vi "tm_setmultiregion_40.vi"(8 "error in (no error)":errorcluster, 10 "Sub Regions":T1(array[cluster]), 11 "Handle in":u32) -> (0 "error out":errorcluster, 3 "Handle out":u32)   [LabVIEW 2023]
uses:
  tmcamcon.dll
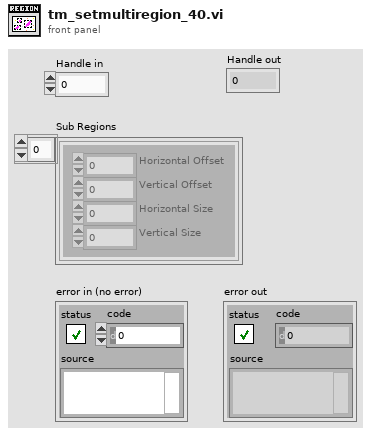
[diagram p1: front panel]
types:
  T1 = cluster{"Horizontal Offset":i32, "Vertical Offset":i32, "Horizontal Size":i32, "Vertical Size":i32}[]
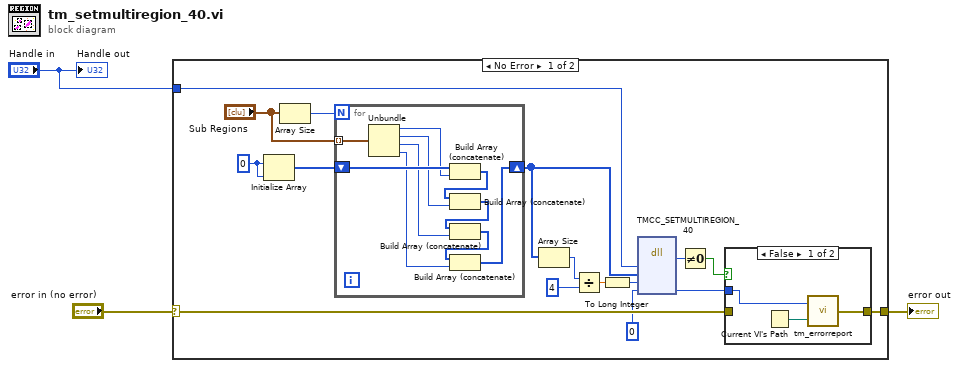
[diagram p0: block diagram]
diagram:
  n1 = case shown="No Error" "error in (no error)" {
    selector: "error in (no error)" -> [w17 w34]
    tunnel: [w14 w34] -> w2
    tunnel: "Handle in" -> [w18 _]
    frame No Error {
      w11 = 0 ("element")
      n2 = Initialize Array(w11, w11) -> (w10:i32[])
      n3 = Array Size(array="Sub Regions") -> (size(s)=w13:i32)
      n4 = for {
        N: w13 -> [_]
        tunnel: "Sub Regions" -> [w29] mode=indexing
        shift-right: [w20] -> w9
        shift-left: w10 -> [w28]
        n5 = Unbundle(w29) -> ("Horizontal Offset"=w27:i32, "Vertical Offset"=w26:i32, "Horizontal Size"=w21:i32, "Vertical Size"=w22:i32)
        n6 = Build Array (concatenate)(w28, w27) -> (w25:i32[])
        n7 = Build Array (concatenate)(w25, w26) -> (w24:i32[])
        n8 = Build Array (concatenate)(w24, w21) -> (w23:i32[])
        n9 = Build Array (concatenate)(w23, w22) -> (w20:i32[])
      }
      n10 = Array Size(array=w9) -> (size(s)=w7:i32)
      n11 = Divide(x=w7, y=4) -> (x/y=w4:dbl)
      n12 = To Long Integer(number=w4) -> (32bit integer=w5:i32)
      n13 = dll-call lib="tmcamcon.dll" fn="TMCC_SETMULTIREGION_40"("HDCAM"=w18, "regionarray"=w9, "totalregions"=w5, "Erval"=0) -> ("return type"=w19:u32, "Erval"=w16:i32)  [unwired: 6 in, 2 out]
      n14 = Not Equal To 0?(x=w19) -> (x != 0?=w15:bool)
      n15 = case shown="False" w15 {
        tunnel: w17 -> [_ w33]
        tunnel: [w31 w33] -> w14
        tunnel: w16 -> [w30 _]
        frame False {
          n16 = Current VI's Path() -> (path=w32:path)
          n17 = call "tm_errorreport.vi"("Source"=w32, "Error"=w30) -> ("error out"=w31:errorcluster)
        }
        frame True {
        }
      }
    }
    frame Error {
    }
  }
  "error out" <- w2
  "Handle out" <- "Handle in"
